vi "Spring Length.vi"(10 "Measured Tension":dbl[](array[numeric]), 11 "Cable Length in":dbl[](array[numeric])) -> (3 "Cable Length out":dbl[](array[numeric]))   [LabVIEW 2021]
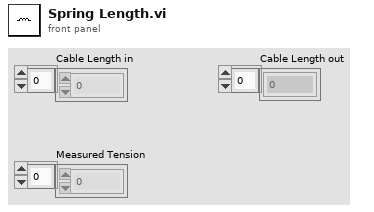
[diagram p1: front panel]
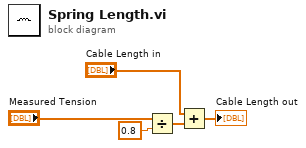
[diagram p0: block diagram]
diagram:
  n1 = Divide(x="Measured Tension", y=0.8) -> (x/y=w4:dbl[])
  n2 = Add(x="Cable Length in", y=w4) -> (x+y=→"Cable Length out":dbl[])
